vi "ModbusMaster.vi"() -> ()   [LabVIEW 2020]
uses:
  <vilib>/NI/Modbus Library/API/Wrapper/Create TCP Master.vi
  <vilib>/NI/Modbus Library/API/Master/Modbus Master.lvclass
  <vilib>/NI/Modbus Library/API/Wrapper/API Main.lvlib
panel:
  in  "stop":bool
  in  "Array":u16[](array[slide]) scale=0.0..100.0
  in  "Coils":bool[](array[boolean])
  # "Modbus Slave"
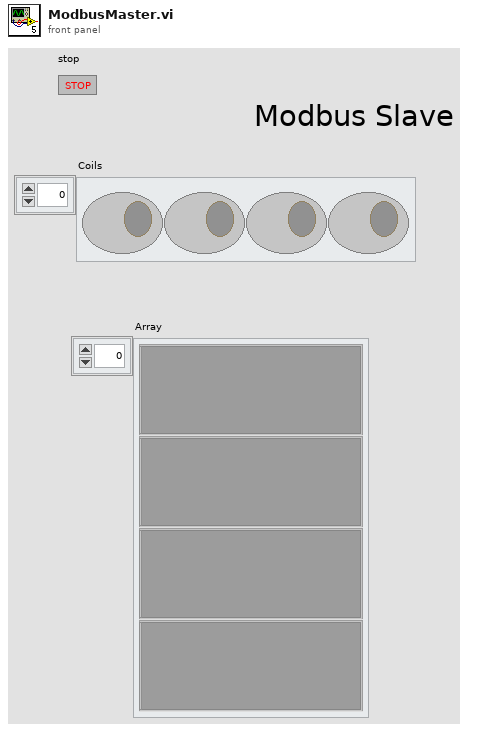
[diagram p1: front panel]
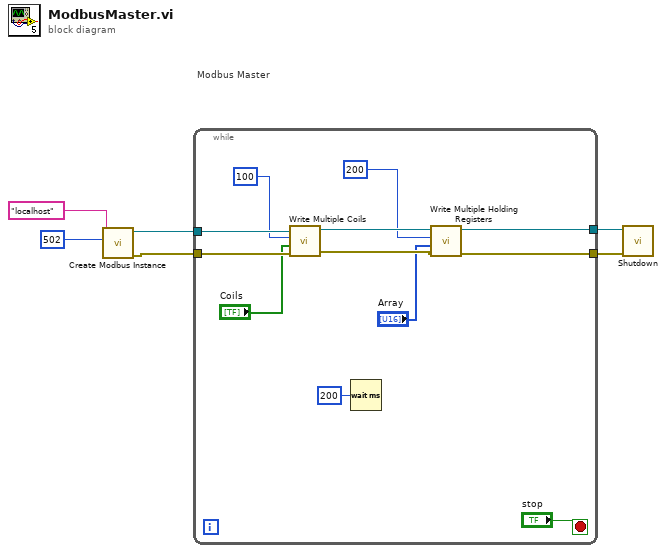
[diagram p0: block diagram]
diagram:
  # "Modbus Master"
  n1 = call-poly <vilib>:"Create Modbus Instance.vi"("port (502)"=u16 502, "address"="localhost") -> ("error out"=w1:errorcluster, "TCP master instance"=w4:refnum<class "Modbus Master.lvclass">)  [unwired: 8 in]
  n2 = while {
    tunnel: w4 -> [w17]
    tunnel: [w15] -> w3
    tunnel: [w14] -> w2
    tunnel: w1 -> [w12]
    stop <- "stop" stop-if-true
    n3 = call-dynamic "Write Multiple Coils.vi"("error in"=w12, "coils to write"="Coils", "starting address"=u16 100, "Modbus master in"=w17) -> ("error out"=w13:errorcluster, "Modbus master out"=w16:refnum<class "Modbus Master.lvclass">)  [unwired: 6 in]
    n4 = Wait (ms)(milliseconds to wait=u32 200) -> ()  [unwired: 1 out]
    n5 = call-dynamic "Write Multiple Holding Registers.vi"("error in"=w13, "registers to write"="Array", "starting address"=u16 200, "Modbus master in"=w16) -> ("error out"=w14:errorcluster, "Modbus master out"=w15:refnum<class "Modbus Master.lvclass">)  [unwired: 6 in]
  }
  n6 = call-dynamic "Shutdown.vi"("error in"=w2, "Modbus master in"=w3) -> ()  [unwired: 9 in, 1 out]
